vi "_Destroy.vi"(8 "error in (no error)":errorcluster, 11 "Collection in":refnum<class "Collection.lvclass">) -> (0 "error out":errorcluster)   [LabVIEW 2023, in "Collection.lvclass"]
uses:
  Collection.lvclass
  Collection.lvclass/Collection.ctl
  Readable/Readable.lvclass
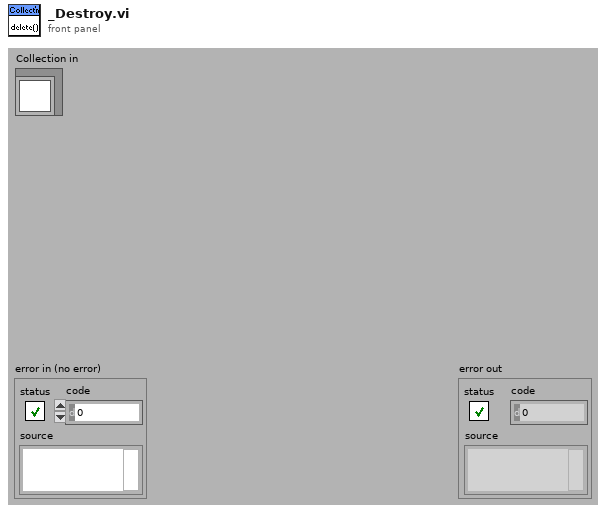
[diagram p1: front panel]
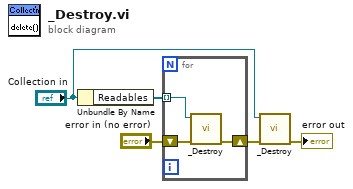
[diagram p0: block diagram]
diagram:
  n1 = Unbundle By Name("Collection in") -> ("Readables"=w5:refnum<class "Readable.lvclass">[])
  n2 = for {
    tunnel: w5 -> [w6] mode=indexing
    shift-right: [w7] -> w4
    shift-left: "error in (no error)" -> [w8]
    n3 = call-dynamic "_Destroy.vi"("error in (no error)"=w8, "Instrument in"=w6) -> ("error out"=w7:errorcluster)  [unwired: 9 out]
  }
  n4 = call-parent "_Destroy.vi"("error in (no error)"=w4, "Instrument in"="Collection in") -> ("error out"=→"error out":errorcluster)  [unwired: 9 out]
